vi "Read_WF_Dataset.vi"(10 "Test dataset path":path=path "D:/Ngene/Projects_SVN/DeepLTK/Examples/2_Waveform_Processing/24_Power_Transmission_Line_Fault_Classification/Dataset/Test", 11 "Train dataset path":path=path "D:/Ngene/Projects_SVN/DeepLTK/Examples/2_Waveform_Processing/24_Power_Transmission_Line_Fault_Classification/Dataset/Train") -> (3 "NN_Dataset":T1={"Train"={"Inputs Ref."=variant(refnum<data-value> refnum), "Outputs Ref."=refnum, "Dims_In"=500, "Dataset_Size"=9000, "Dims_Out"=6, "Labels"=["DC Offset", "Interruption", "Normal", "Sag", "Swell", "Transient"], "File Paths"=[]}, "Validation"={"Inputs Ref."=variant(refnum<data-value> refnum), "Outputs Ref."=refnum, "Dims_In"=0, "Dataset_Size"=0, "Dims_Out"=0, "Labels"=[], "File Paths"=[]}, "Test"={"Inputs Ref."=variant(refnum<data-value> refnum), "Outputs Ref."=refnum, "Dims_In"=500, "Dataset_Size"=1800, "Dims_Out"=6, "Labels"=["DC Offset", "Interruption", "Normal", "Sag", "Swell", "Transient"], "File Paths"=[]}})   [LabVIEW 2020]
uses:
  <vilib>/Ngene/Deep Learning Toolkit/Toolkit/NN_Data/API/DataSet/DataSet_Types/NN_DataSets_All(In1D_Out1D).ctl
  <vilib>/Ngene/Deep Learning Toolkit/Toolkit/NN_Data/API/DataSet/DataSet_Types/NN_DataSet(In1D_Out1D).ctl
  <vilib>/Ngene/Deep Learning Toolkit/Toolkit/NN_Data/Controls/DataRef_Types/2D/NN_Data_ref(2D_SGL).ctl
  <vilib>/Utility/file.llb/Read Delimited Spreadsheet (DBL).vi
  <vilib>/Ngene/Deep Learning Toolkit/Toolkit/Deep_Learning_Toolkit_by_Ngene.lvlib
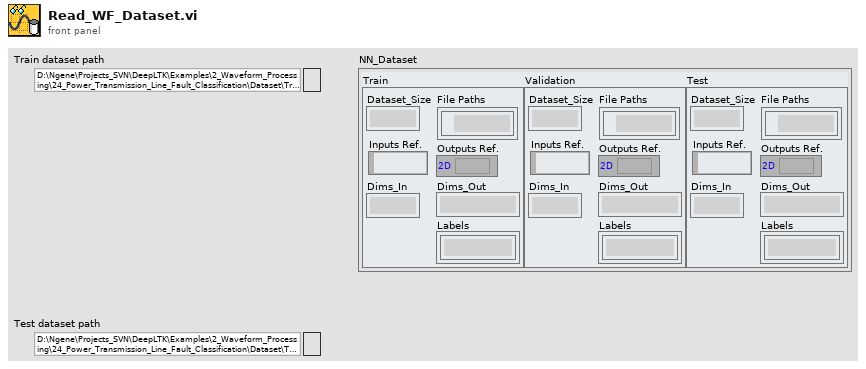
[diagram p1: front panel]
types:
  T1 = typedef "Deep_Learning_Toolkit_by_Ngene.lvlib/NN_DataSets_All(In1D_Out1D).ctl" = cluster{"Train":T2, "Validation":T2, "Test":T2}
  T2 = typedef "Deep_Learning_Toolkit_by_Ngene.lvlib/NN_DataSet(In1D_Out1D).ctl" = cluster{"Inputs Ref.":variant, "Outputs Ref.":T3, "Dims_In":i32, "Dataset_Size":i32, "Dims_Out":i32, "Labels":string[], "File Paths":path[]}
  T3 = typedef "Deep_Learning_Toolkit_by_Ngene.lvlib/NN_Data_ref(2D_SGL).ctl" = refnum<data-value>
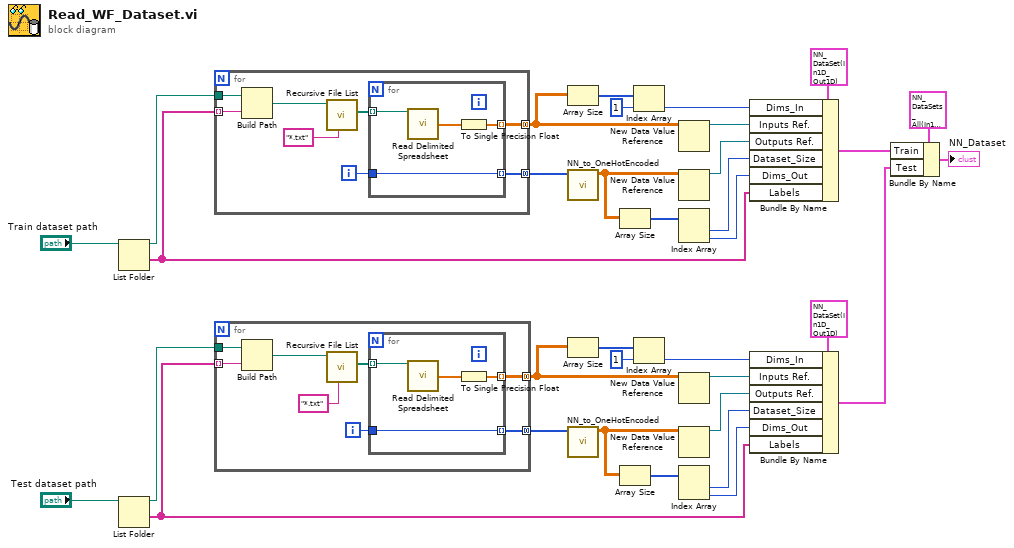
[diagram p0: block diagram]
diagram:
  n1 = List Folder(path="Train dataset path") -> (path out=w34:path, folder names=w22:string[])  [unwired: 3 in, 2 out]
  n2 = List Folder(path="Test dataset path") -> (path out=w6:path, folder names=w18:string[])  [unwired: 3 in, 2 out]
  n3 = for {
    tunnel: w34 -> [w42]
    tunnel: w22 -> [w35] mode=indexing
    tunnel: [w36] -> w2 mode=concatenating
    tunnel: [w37] -> w3 mode=concatenating
    i -> [w38]
    n4 = Build Path(base path=w42, name or relative path=w35) -> (appended path=w41:path)
    n5 = call <vilib>:"Recursive File List.vi"("pattern"="*.txt", "Folder Path"=w41) -> ("All Files in Dir"=w39:path[])  [unwired: 5 in, 4 out]
    n6 = for {
      tunnel: w39 -> [w46] mode=indexing
      tunnel: [w44] -> w36 mode=indexing
      tunnel: w38 -> [w43]
      tunnel: [w43] -> w37 mode=indexing
      n7 = call-poly <vilib>:"Read Delimited Spreadsheet.vi"("file path (dialog if empty)"=w46) -> ("first row"=w45:dbl[])  [unwired: 9 in, 5 out]
      n8 = To Single Precision Float(number=w45) -> (single precision float=w44:sgl[])
    }
  }
  n9 = for {
    tunnel: w6 -> [w54]
    tunnel: w18 -> [w47] mode=indexing
    tunnel: [w48] -> w1 mode=concatenating
    tunnel: [w49] -> w4 mode=concatenating
    i -> [w50]
    n10 = Build Path(base path=w54, name or relative path=w47) -> (appended path=w53:path)
    n11 = call <vilib>:"Recursive File List.vi"("pattern"="*.txt", "Folder Path"=w53) -> ("All Files in Dir"=w51:path[])  [unwired: 5 in, 4 out]
    n12 = for {
      tunnel: w51 -> [w58] mode=indexing
      tunnel: [w56] -> w48 mode=indexing
      tunnel: w50 -> [w55]
      tunnel: [w55] -> w49 mode=indexing
      n13 = call-poly <vilib>:"Read Delimited Spreadsheet.vi"("file path (dialog if empty)"=w58) -> ("first row"=w57:dbl[])  [unwired: 9 in, 5 out]
      n14 = To Single Precision Float(number=w57) -> (single precision float=w56:sgl[])
    }
  }
  n15 = Array Size(array=w2) -> (size(s)=w30:i32[])
  n16 = call <vilib>:"NN_to_OneHotEncoded.vi"("Label_Idx"=w3) -> ("Prediction"=w26:sgl[][])  [unwired: 10 in]
  n17 = Array Size(array=w1) -> (size(s)=w10:i32[])
  n18 = call <vilib>:"NN_to_OneHotEncoded.vi"("Label_Idx"=w4) -> ("Prediction"=w14:sgl[][])  [unwired: 10 in]
  n19 = Array Size(array=w26) -> (size(s)=w25:i32[])
  n20 = Array Size(array=w14) -> (size(s)=w15:i32[])
  n21 = Index Array(array=w30, index=1) -> (element=w29:i32)
  n22 = Index Array(array=w10, index=1) -> (element=w11:i32)
  n23 = New Data Value Reference(data value=w2) -> (data value reference=w28:refnum<data-value>)  [unwired: 1 in, 1 out]
  n24 = New Data Value Reference(data value=w26) -> (data value reference=w27:refnum<data-value>)  [unwired: 1 in, 1 out]
  n25 = Index Array(array=w25) -> (element #1=w24:i32, element #2=w23:i32)  [unwired: 2 in]
  n26 = New Data Value Reference(data value=w1) -> (data value reference=w12:refnum<data-value>)  [unwired: 1 in, 1 out]
  n27 = New Data Value Reference(data value=w14) -> (data value reference=w13:refnum<data-value>)  [unwired: 1 in, 1 out]
  n28 = Index Array(array=w15) -> (element #1=w16:i32, element #2=w17:i32)  [unwired: 2 in]
  n29 = Bundle By Name(cluster=T2 {"Inputs Ref."=variant(refnum<data-value> refnum), "Outputs Ref."=refnum, "Dims_In"=0, "Dataset_Size"=0, "Dims_Out"=0, "Labels"=[], "File Paths"=[]} ("Dataset(In1D_Out1D)"), "Dims_In"=w29, "Inputs Ref."=w28, "Outputs Ref."=w27, "Dataset_Size"=w24, "Dims_Out"=w23, "Labels"=w22) -> (w21:T2)
  n30 = Bundle By Name(cluster=T2 {"Inputs Ref."=variant(refnum<data-value> refnum), "Outputs Ref."=refnum, "Dims_In"=0, "Dataset_Size"=0, "Dims_Out"=0, "Labels"=[], "File Paths"=[]} ("Dataset(In1D_Out1D)"), "Dims_In"=w11, "Inputs Ref."=w12, "Outputs Ref."=w13, "Dataset_Size"=w16, "Dims_Out"=w17, "Labels"=w18) -> (w5:T2)
  n31 = Bundle By Name(cluster=T1 {"Train"={"Inputs Ref."=variant(refnum<data-value> refnum), "Outputs Ref."=refnum, "Dims_In"=0, "Dataset_Size"=0, "Dims_Out"=0, "Labels"=[], "File Paths"=[]}, "Validation"={"Inputs Ref."=variant(refnum<data-value> refnum), "Outputs Ref."=refnum, "Dims_In"=0, "Dataset_Size"=0, "Dims_Out"=0, "Labels"=[], "File Paths"=[]}, "Test"={"Inputs Ref."=variant(refnum<data-value> refnum), "Outputs Ref."=refnum, "Dims_In"=0, "Dataset_Size"=0, "Dims_Out"=0, "Labels"=[], "File Paths"=[]}} ("Datasets_All(In1D_Out1D)"), "Train"=w21, "Test"=w5) -> (→"NN_Dataset":T1)
